vi "Project4_Gcode.vi"() -> ()   [LabVIEW 2024]
uses:
  <userlib>/SerialVIs/subs/portX.xctl
panel:
  out "reply":string
  in  "portX 2":refnum<visa-resource-name>(xcontrol)
  out "Bot Arm 2":picture
  out "Angle 2":dbl
  out "Angle 1":dbl
  in  "Colors 2":T1={"Base"=16750848, "Link 1"=16764006, "Joint 2"=26316, "Link 2"=6723993, "EOF"=16724787}
  out "GCode Reading":picture
  in  "file (use dialog)":path
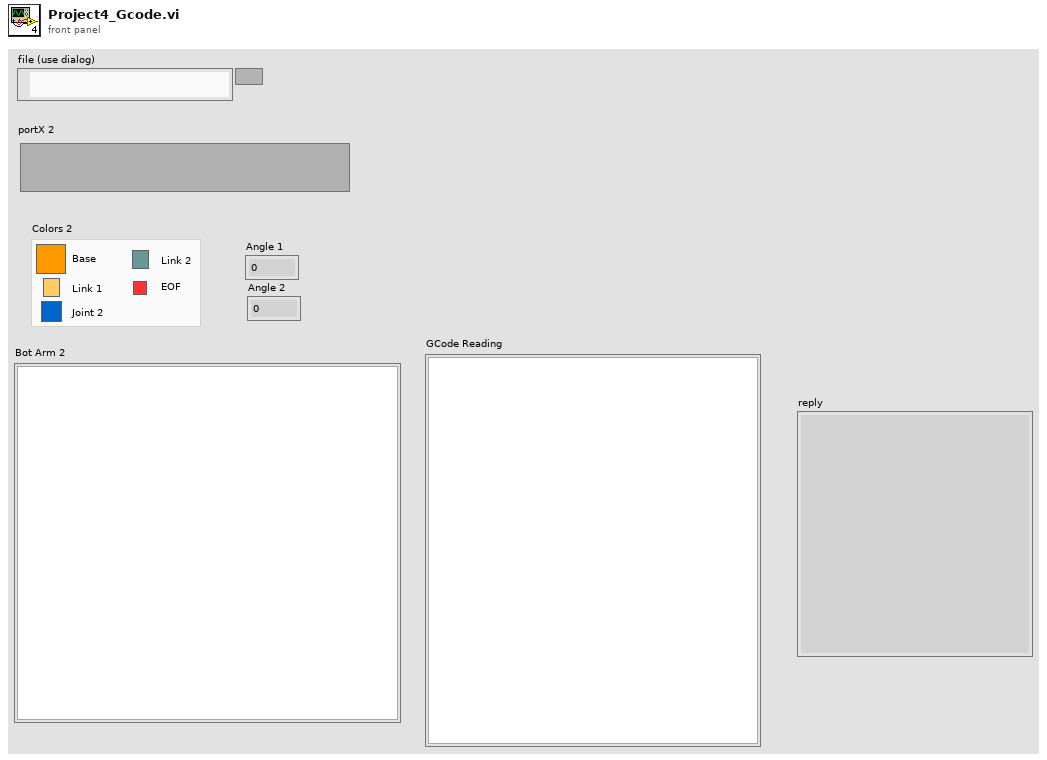
[diagram p1: front panel]
types:
  T1 = cluster{"Base":u32, "Link 1":u32, "Joint 2":u32, "Link 2":u32, "EOF":u32}
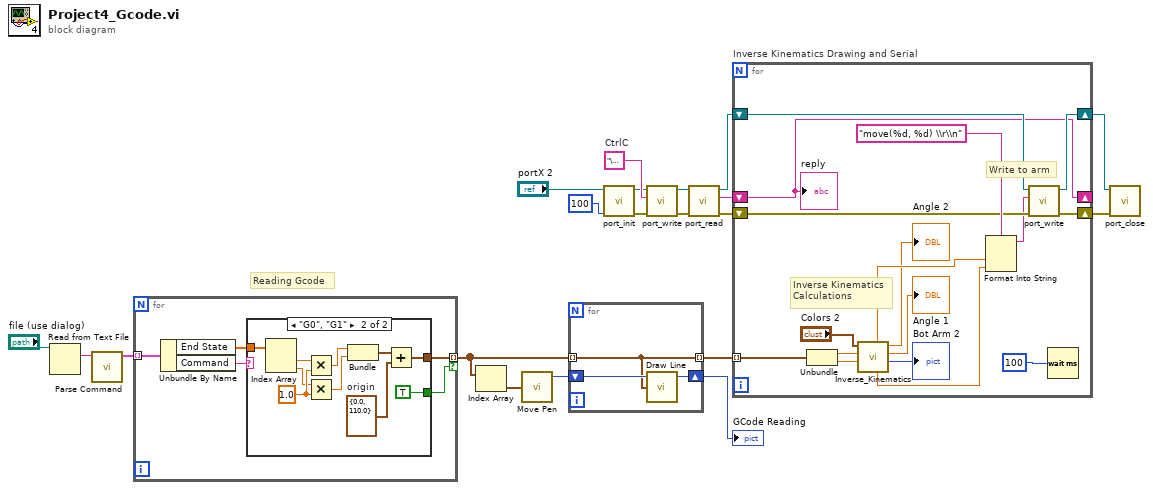
[diagram p0: block diagram]
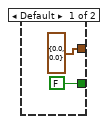
[diagram p2: hidden frame]
diagram:
  w12 = "\u0003"  # CtrlC
  # "Reading Gcode"
  n1 = Read from Text File(file (use dialog)="file (use dialog)") -> (text=w19:string)  [unwired: 3 in, 3 out]
  n2 = call "Parse Command.vi"("text"=w19) -> ("cmd amd State"=w18:cluster{"Command":string, "End State":dbl[]}[])  [unwired: 8 in, 2 out]
  n3 = for {
    tunnel: w18 -> [w25] mode=indexing
    tunnel: [w22] -> w14 mode=indexing if=w21
    n4 = Unbundle By Name(w25) -> ("End State"=w23:dbl[], "Command"=w24:string)
    n5 = case shown="\"G0\", \"G1\"" w24 {
      tunnel: w23 -> [_ w37]
      tunnel: [cluster{dbl, dbl} {0.0, 0.0} w34] -> w22
      tunnel: [FALSE TRUE] -> w21
      frame Default {
      }
      frame "G0", "G1" {
        w32 = 1.0 ("y")
        w35 = cluster{dbl, dbl} {0.0, 110.0}  # origin
        n6 = Index Array(array=w37) -> (element #1=w29:dbl, element #2=w28:dbl)  [unwired: 2 in]
        n7 = Multiply(x=w29, y=w32) -> (x*y=w30:dbl)
        n8 = Multiply(x=w28, y=w32) -> (x*y=w31:dbl)
        n9 = Bundle(w30, w31) -> (w36:cluster{dbl, dbl})  [unwired: 1 in]
        n10 = Add(x=w36, y=w35) -> (x+y=w34:cluster{dbl, dbl})
      }
    }
  }
  n11 = Index Array(array=w14) -> (element=w17:cluster{dbl, dbl})  [unwired: 1 in]
  n12 = call <vilib>:"Move Pen.vi"("new position"=w17) -> ("new picture"=w16:picture)  [unwired: 4 in]
  n13 = for {
    shift-right: [w39] -> w15
    shift-left: w16 -> [w40]
    tunnel: w14 -> [w38] mode=indexing
    tunnel: [w38] -> w13 mode=indexing
    n14 = call <vilib>:"Draw Line.vi"("picture"=w40, "end point"=w38) -> ("new picture"=w39:picture)  [unwired: 7 in]
  }
  "GCode Reading" <- w15
  n15 = call <userlib>:"port_init.vi"("Timeout (ms)"=u32 100, "VISA Refnum in"="portX 2") -> ("error out"=w10:errorcluster, "VISA Refnum out"=w11:refnum<visa-resource-name>)  [unwired: 8 in]
  n16 = call <userlib>:"port_write.vi"("error in (no error)"=w10, "write buffer"=w12, "VISA Refnum in"=w11) -> ("error out"=w8:errorcluster, "VISA Refnum out"=w9:refnum<visa-resource-name>)  [unwired: 7 in]
  n17 = call <userlib>:"port_read.vi"("error in (no error)"=w8, "VISA Refnum in"=w9) -> ("error out"=w4:errorcluster, "reply"=w3:string, "VISA Refnum out"=w5:refnum<visa-resource-name>)  [unwired: 7 in]
  n18 = for "Inverse Kinematics Drawing and Serial" {
    tunnel: w13 -> [w54] mode=indexing
    shift-right: [w44] -> _
    shift-left: w3 -> [w44]
    shift-right: [w46] -> w2
    shift-left: w5 -> [w48]
    shift-right: [w45] -> w1
    shift-left: w4 -> [w47]
    # "Write to arm"
    # "Inverse Kinematics\nCalculations"
    n19 = Unbundle(w54) -> (w53:dbl, w52:dbl)
    n20 = call "Inverse_Kinematics.vi"("Numeric in"=w52, "Numeric 3"=w53, "Colors in"="Colors 2") -> ("Picture Out"=→"Bot Arm 2":picture, "Angle 3"=→"Angle 1":dbl, "Angle 4"=→"Angle 2":dbl, "angle2"=w49:dbl, "Numeric out"=w50:dbl)  [unwired: 4 in]
    n21 = Format Into String(format string="move(%d, %d) \\r\\n", w50, w49) -> (resulting string=w43:string)  [unwired: 2 in, 1 out]
    n22 = call <userlib>:"port_write.vi"("error in (no error)"=w47, "write buffer"=w43, "VISA Refnum in"=w48) -> ("error out"=w45:errorcluster, "VISA Refnum out"=w46:refnum<visa-resource-name>)  [unwired: 7 in]
    n23 = Wait (ms)(milliseconds to wait=u32 100) -> ()  [unwired: 1 out]
    "reply" <- w44
  }
  n24 = call <userlib>:"port_close.vi"("error in (no error)"=w1, "VISA Refnum in"=w2) -> ()  [unwired: 10 in]
